vi "Image-smoothing.vi"(8 "error in":errorcluster, 9 "Correct. params. ref. in":refnum<data-value>, 10 "Buffer element in":T1 {"Temperature characteristics"."Stand. dev. temperature" format="%#.1f"; "Temperature characteristics"."Min. temperature" format="%#.0f"; "Temperature characteristics"."Max. temperature" format="%#.0f"; "Temperature characteristics"."Average temperature" format="%#.0f"}) -> (0 "error IO":errorcluster, 1 "Correct. params. ref.":refnum<data-value>, 2 "Buffer element":T1 {"Temperature characteristics"."Stand. dev. temperature" format="%#.1f"; "Temperature characteristics"."Min. temperature" format="%#.0f"; "Temperature characteristics"."Max. temperature" format="%#.0f"; "Temperature characteristics"."Average temperature" format="%#.0f"})   [LabVIEW 2013, in "CameraVision.lvlib" / "CV-Main.lvclass"]
uses:
  CV-Main.lvclass
  Buffers/Storage-buffer.ctl
  <vilib>/vision/Image Controls.llb/IMAQ Image.ctl
  Temperature/Temperature-characteristics.ctl
  Analysis/Characteristics-cluster.ctl
  Correction/CV-Correction.lvclass
  Correction/CV-Correction.lvclass/CV-Correction.ctl
  Correction/Read Threshold only 2nd camera image.vi
  Correction/Read Always threshold when smoothing.vi
  Correction/Read Median filter type.vi
  Correction/Read Gaussian filter kernel size.vi
  Correction/Read Gaussian filter kernel number.vi
  Correction/Read Noise treshold.vi
  Correction/Read Smoothing algorithm.vi
  Correction/Read Image smoothing.vi
  Temperature/CV-Temperature.lvclass
  Analysis/CV-Analysis.lvclass
  Buffers/CV-Buffers.lvclass
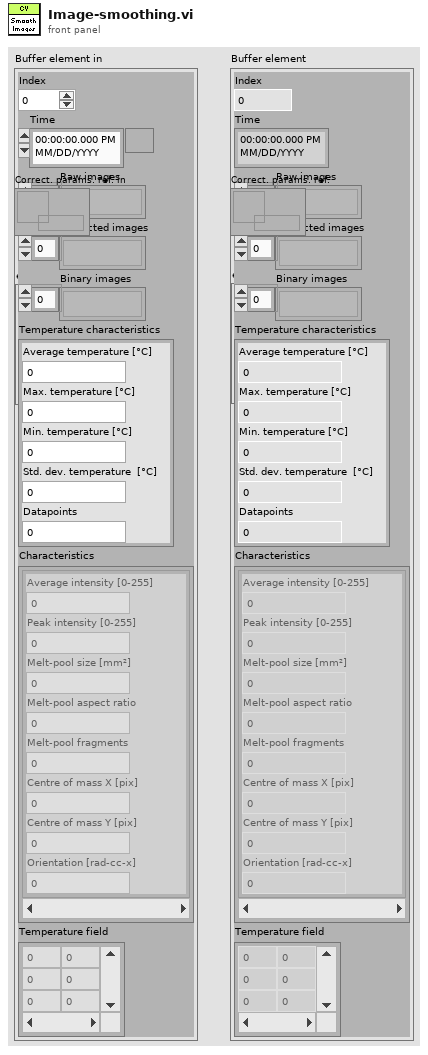
[diagram p1: front panel]
types:
  T1 = typedef "CameraVision.lvlib/CV-Buffers.lvclass/Storage-buffer.ctl" = cluster{"Index":i32, "Time":timestamp, "Raw images":T2[], "Corrected images":T2[], "Binary images":T2[], "Temperature characteristics":T3, "Characteristics":T4[], "Temperature field":dbl[][]}
  T2 = typedef "IMAQ Image.ctl" = refnum<image>
  T3 = typedef "CameraVision.lvlib/CV-Temperature.lvclass/Temperature-characteristics.ctl" = cluster{"Average temperature ":dbl, "Max. temperature":dbl, "Min. temperature":dbl, "Stand. dev. temperature":dbl, "Datapoints":dbl}
  T4 = typedef "CameraVision.lvlib/CV-Analysis.lvclass/Characteristics-cluster.ctl" = cluster{"Average intensity":dbl, "Peak intensity":dbl, "Melt-pool size":dbl, "Melt-pool aspect ratio":dbl, "Melt-pool fragments":dbl, "Centre of mass X":dbl, "Centre of mass Y":dbl, "Orientation":dbl}
  T5 = cluster{"X Size":i32, "Y Size":i32, "Order #":i32}
  T6 = typedef "CameraVision.lvlib/CV-Correction.lvclass/Smoothing.ctl" = enum16{"Noise tresholding", "NT+Median filter", "NT+Gaussian filter"}
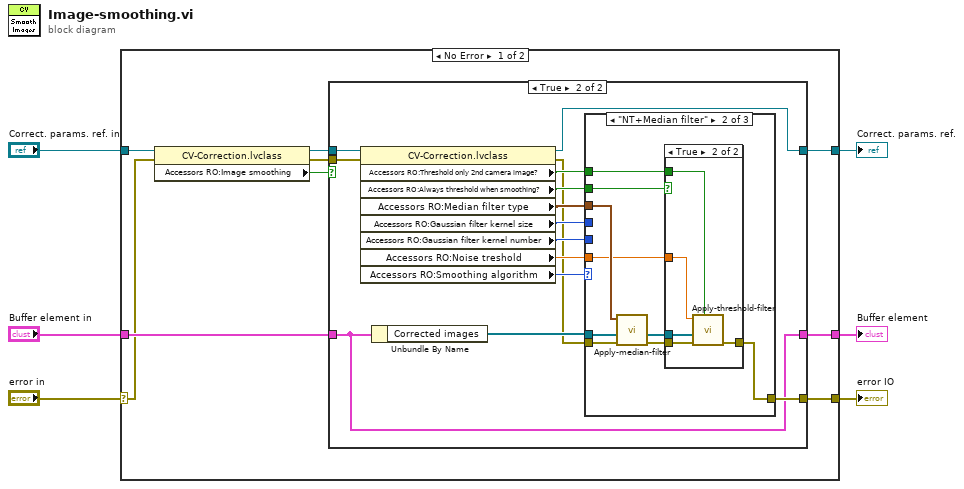
[diagram p0: block diagram]
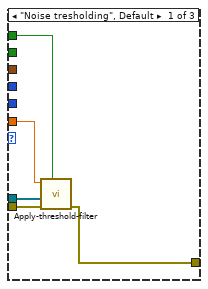
[diagram p3: hidden frame]
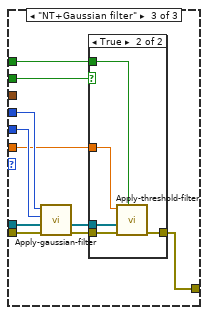
[diagram p5: hidden frame]
diagram:
  n1 = case shown="No Error" "error in" {
    selector: "error in" -> [w9 w69]
    tunnel: "Correct. params. ref. in" -> [w13 w68]
    tunnel: [w15 w69] -> w6
    tunnel: "Buffer element in" -> [w14 w67]
    tunnel: [w8 w68] -> w3
    tunnel: [w7 w67] -> w1
    frame No Error {
      n2 = property class="CV-Correction.lvclass"(reference=w13, error in=w9) -> (reference out=w12:refnum<data-value>, error out=w10:errorcluster, "Accessors RO:Image smoothing"=w11:bool)
      n3 = case shown="True" w11 {
        tunnel: w12 -> [w17 w23]
        tunnel: [w18 w32] -> w15
        tunnel: w14 -> [w16 w19]
        tunnel: w10 -> [w18 w22]
        tunnel: [w17 w20] -> w8
        tunnel: [w16 w19] -> w7
        frame False {
        }
        frame True {
          n4 = property class="CV-Correction.lvclass"(reference=w23, error in=w22) -> (reference out=w20:refnum<data-value>, error out=w21:errorcluster, "Accessors RO:Threshold only 2nd camera image?"=w30:bool, "Accessors RO:Always threshold when smoothing?"=w29:bool, "Accessors RO:Median filter type"=w28:T5, "Accessors RO:Gaussian filter kernel size"=w27:i32, "Accessors RO:Gaussian filter kernel number"=w26:i32, "Accessors RO:Noise treshold"=w25:sgl, "Accessors RO:Smoothing algorithm"=w24:T6)
          n5 = Unbundle By Name(w19) -> ("Corrected images"=w31:T2[])
          n6 = case shown="\"NT+Median filter\"" w24 {
            tunnel: [w36 w45 w52] -> w32
            tunnel: w31 -> [w35 w40 w55]
            tunnel: w21 -> [w37 w44 w60]
            tunnel: w25 -> [w34 w38 w54]
            tunnel: w30 -> [w33 w39 w57]
            tunnel: w29 -> [_ w41 w53]
            tunnel: w28 -> [_ w42 _]
            tunnel: w27 -> [_ _ w59]
            tunnel: w26 -> [_ _ w58]
            frame "Noise tresholding", Default {
              n7 = call "Apply-threshold-filter.vi"("Threshold only 2nd camera image?"=w33, "error in"=w37, "Corrected"=w35, "Noise treshold"=w34) -> ("error IO"=w36:errorcluster)  [unwired: 7 in]
            }
            frame "NT+Median filter" {
              n8 = call "Apply-median-filter.vi"("error in"=w44, "Corrected"=w40, "Median filter type"=w42) -> ("error IO"=w43:errorcluster)  [unwired: 8 in]
              n9 = case shown="True" w41 {
                tunnel: [w46 w51] -> w45
                tunnel: w43 -> [w46 w50]
                tunnel: w40 -> [_ w49]
                tunnel: w39 -> [_ w48]
                tunnel: w38 -> [_ w47]
                frame False {
                }
                frame True {
                  n10 = call "Apply-threshold-filter.vi"("Threshold only 2nd camera image?"=w48, "error in"=w50, "Corrected"=w49, "Noise treshold"=w47) -> ("error IO"=w51:errorcluster)  [unwired: 7 in]
                }
              }
            }
            frame "NT+Gaussian filter" {
              n11 = call "Apply-gaussian-filter.vi"("error in"=w60, "Corrected"=w55, "Kernel Number"=w58, "Kernel Size"=w59) -> ("error IO"=w56:errorcluster)  [unwired: 7 in]
              n12 = case shown="True" w53 {
                tunnel: [w61 w66] -> w52
                tunnel: w56 -> [w61 w65]
                tunnel: w55 -> [_ w64]
                tunnel: w57 -> [_ w63]
                tunnel: w54 -> [_ w62]
                frame False {
                }
                frame True {
                  n13 = call "Apply-threshold-filter.vi"("Threshold only 2nd camera image?"=w63, "error in"=w65, "Corrected"=w64, "Noise treshold"=w62) -> ("error IO"=w66:errorcluster)  [unwired: 7 in]
                }
              }
            }
          }
        }
      }
    }
    frame Error {
    }
  }
  "error IO" <- w6
  "Buffer element" <- w1
  "Correct. params. ref." <- w3
